vi "Teleop.vi"(10 "Match Info":T1={"Autonomous Elapsed Seconds"=0.0, "TeleOp Elapsed Seconds"=0.0, "Disabled Elapsed Seconds"=0.0, "Visited Autonomous"=FALSE, "Visited TeleOp"=FALSE, "Visited Disabled"=FALSE, "Autonomous Settings"={"Autonomous Style"=enum."Independent", "VI Refnum"=refnum}}, 11 "Call Context":T2) -> ()   [LabVIEW 2014]
doc: "This VI is called for each TeleOp packet received from the DS where the robot is not disabled. It is often used to read from the joysticks and update I/O or to update setpoints for timed control loops. It should complete and return within 20 milliseconds or it may miss DS packets."
uses:
  <vilib>/Rock Robotics/WPI/DriverStation/WPI_DriverStationDerivedRobotMode.ctl
  <vilib>/Rock Robotics/WPI/DriverStation/WPI_DriverStationMatch Info.ctl
  <vilib>/Rock Robotics/Network Tables/SD Read Boolean.vi
  <vilib>/Rock Robotics/Network Tables/SD Read Number.vi
  <vilib>/Rock Robotics/WPI/RobotDrive/WPI_RobotDriveGetSetRefNum.vi
  <vilib>/Rock Robotics/WPI/Joystick/WPI_JoystickGetSetRefNum.vi
  <vilib>/Rock Robotics/Network Tables/SD Write Boolean Array.vi
  <vilib>/Rock Robotics/Network Tables/SD Write Numeric Array.vi
  <vilib>/Rock Robotics/WPI/Solenoid/Deprecated/WPI_SolenoidSetBool.vi
panel:
  in  "Numeric":dbl
  out "2":dbl
  out "9":dbl
  out "8":dbl
  out "Sample Slider 0":dbl(slide) scale=0.0..5.0
  out "Sample Boolean 1":bool
  out "Sample Boolean 0":bool
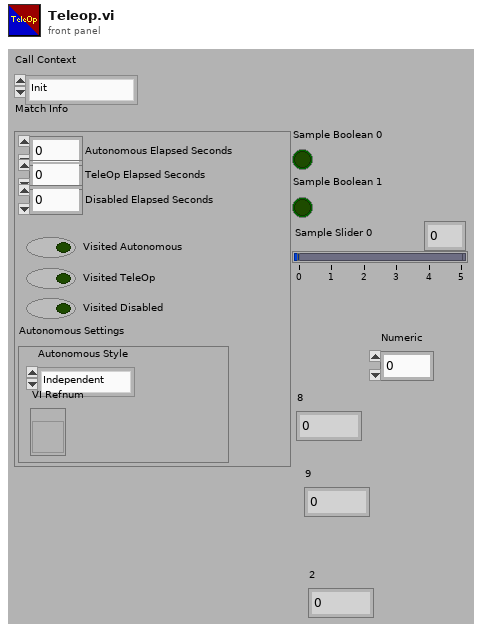
[diagram p1: front panel]
types:
  T1 = typedef "WPI_DriverStationMatch Info.ctl" = cluster{"Autonomous Elapsed Seconds":dbl, "TeleOp Elapsed Seconds":dbl, "Disabled Elapsed Seconds":dbl, "Visited Autonomous":bool, "Visited TeleOp":bool, "Visited Disabled":bool, "Autonomous Settings":cluster{"Autonomous Style":enum16{"Iterative", "Independent"}, "VI Refnum":refnum<vi>}}
  T2 = typedef "WPI_DriverStationDerivedRobotMode.ctl" = enum16{"Init", "Execute", "Stop"}
  T3 = typedef "WPI_JoystickDevRef.ctl" = cluster{"Device":T4}
  T4 = typedef "WPI_JoystickDeviceEnum.ctl" = enum16{"USB 0", "USB 1", "USB 2", "USB 3", "USB 4", "USB 5"}
  T5 = typedef "WPI_RobotDriveDevRef.ctl" = cluster{"DevStatus":errorcluster, "Motors[]":T6[], "Square Inputs":bool, "Max Output":dbl}
  T6 = typedef "WPI_MotorControlDeviceRef.ctl" = cluster{"DeviceStatus":errorcluster, "Type":T7, "PWM":cluster{"Controller":T8, "PWM Channel":T9, "DeadBand":T10}, "CAN":cluster{"Device Number":u8, "Control Mode":T11, "Semaphore":T12, "Max Vout":dbl, "TalonSRX Control Mode":T13}, "Invert":bool, "TransformRef":T14, "InvTransformRef":T14}
  T7 = typedef "WPI_MotorControlType.ctl" = enum16{"PWM", "CAN", "CANTalonSRX"}
  T8 = typedef "FPGA_TypedefDigitalModule.ctl" = enum16{"Controller 1"}
  T9 = typedef "FPGA_DIOPWMChannel.ctl" = enum8{"PWM 0", "PWM 1", "PWM 2", "PWM 3", "PWM 4", "PWM 5", "PWM 6", "PWM 7", "PWM 8", "PWM 9", "PWM MXP 0", "PWM MXP 1", "PWM MXP 2", "PWM MXP 3", "PWM MXP 4", "PWM MXP 5", "PWM MXP 6", "PWM MXP 7", "PWM MXP 8", "PWM MXP 9", "Invalid"}
  T10 = typedef "WPI_PWMDeadband.ctl" = cluster{"Name":string, "maxPositivePwm":i32, "minPositivePwm":i32, "centerPwm":i32, "maxNegativePwm":i32, "minNegativePwm":i32, "angularRange":u16}
  T11 = typedef "WPI_CANJaguar_ControlMode.ctl" = enum8{"Percent VBus", "Current", "Speed", "Position", "Voltage"}
  T12 = typedef "Semaphore RefNum" = refnum<k1>
  T13 = typedef "WPI_CANTalonSRX_APIControlMode.ctl" = enum8{"Percent VBus", "Speed", "Position", "Slave", "Unchanged / Invalid"}
  T14 = typedef "WPI_PWMTransform_ConPane.ctl" = refnum<vi>
  T15 = cluster{"Buttons[0]":bool, "Buttons[1]":bool, "Buttons[2]":bool, "Buttons[3]":bool, "Buttons[4]":bool, "Buttons[5]":bool, "Buttons[6]":bool, "Buttons[7]":bool, "Buttons[8]":bool}
  T16 = cluster{"Axes[0]":dbl, "Axes[1]":dbl, "Axes[2]":dbl, "Axes[3]":dbl, "Axes[4]":dbl, "Axes[5]":dbl, "Axes[6]":dbl, "Axes[7]":dbl, "Axes[8]":dbl}
  T17 = typedef "WPI_SolenoidDevRef.ctl" = cluster{"DevStatus":errorcluster, "Pneumatics Control Module":u8, "Forward Solenoid Channel":T18, "Reverse Solenoid Channel":T18}
  T18 = typedef "WPI_SolenoidChannel.ctl" = enum8{"Solenoid 0", "Solenoid 1", "Solenoid 2", "Solenoid 3", "Solenoid 4", "Solenoid 5", "Solenoid 6", "Solenoid 7", "Invalid"}
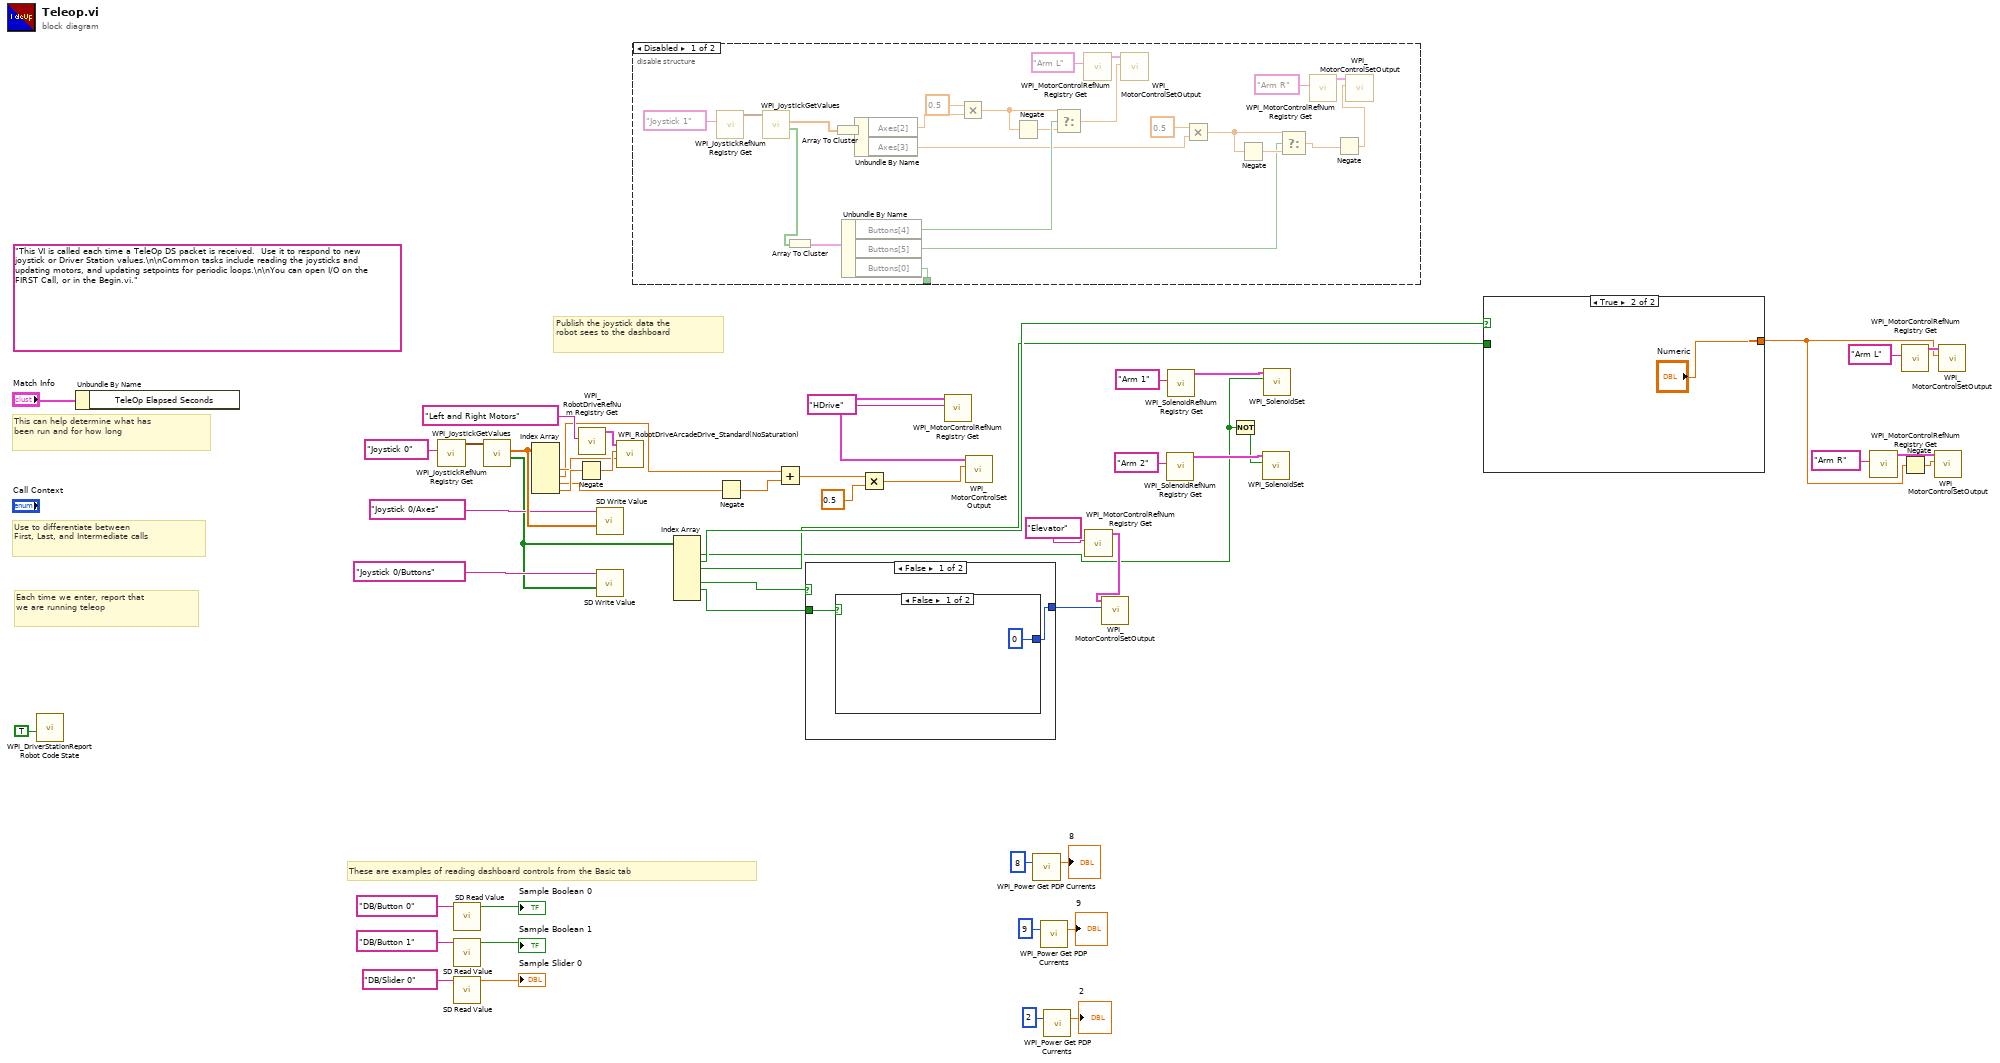
[diagram p0: block diagram]
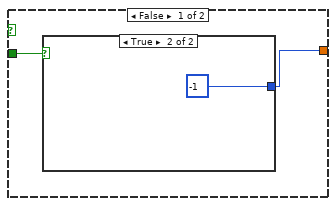
[diagram p3: hidden frame]
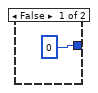
[diagram p4: hidden frame]
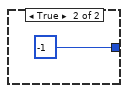
[diagram p5: hidden frame]
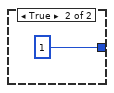
[diagram p6: hidden frame]
diagram:
  (unwired) "This VI is called each time a TeleOp DS packet is received.  Use it to respond to new joystick or Driver Station values.\n\nCommon tasks include reading the joysticks and updating motors, and updating setpoints for periodic loops.\n\nYou can open I/O on the FIRST Call, or in the Begin.vi."
  # "Publish the joystick data the\nrobot sees to the dashboard"
  # "These are examples of reading dashboard controls from the Basic tab"
  # "Each time we enter, report that\nwe are running teleop"
  # "Use to differentiate between\nFirst, Last, and Intermediate calls"
  # "This can help determine what has\nbeen run and for how long"
  n1 = call <vilib>:"WPI_DriverStationReport Robot Code State.vi"("TeleOp"=TRUE ("Autonomous")) -> ()  [unwired: 10 in, 1 out]
  n2 = Unbundle By Name("Match Info") -> ()  [unwired: 1 out]
  n3 = call <vilib>:"WPI_JoystickRefNum Registry Get.vi"("refnum name"="Joystick 0") -> ("JoystickDevRef"=w37:T3)  [unwired: 1 in, 9 out]
  n4 = call-poly <vilib>:"SD Read Value.vi"("Name"="DB/Button 0" ("refnum name")) -> ("Boolean"=→"Sample Boolean 0":bool)  [unwired: 8 in, 2 out]
  n5 = call-poly <vilib>:"SD Read Value.vi"("Name"="DB/Button 1" ("refnum name")) -> ("Boolean"=→"Sample Boolean 1":bool)  [unwired: 8 in, 2 out]
  n6 = call-poly <vilib>:"SD Read Value.vi"("Name"="DB/Slider 0" ("refnum name")) -> ("Numeric"=→"Sample Slider 0":dbl)  [unwired: 8 in, 2 out]
  n7 = call <vilib>:"WPI_JoystickGetValues.vi"("JoystickDevRef"=w37) -> ("Buttons"=w29:bool[], "Axes"=w41:dbl[])  [unwired: 6 in, 3 out]
  n8 = Index Array(array=w41) -> (element #2=w42:dbl, element #3=w33:dbl, element #4=w34:dbl, element #5=w44:dbl)  [unwired: 5 in, 1 out]
  n9 = Negate(x=w44) -> (-x=w43:dbl)
  n10 = call <vilib>:"WPI_RobotDriveRefNum Registry Get.vi"("refnum name"="Left and Right Motors") -> ("RobotDriveDevRef"=w40:T5)  [unwired: 1 in, 9 out]
  n11 = call-poly <vilib>:"SD Write Value.vi"("Numeric Array"=w41, "Name"="Joystick 0/Axes") -> ()  [unwired: 8 in, 2 out]
  n12 = call-poly <vilib>:"SD Write Value.vi"("Boolean Array"=w29, "Name"="Joystick 0/Buttons") -> ()  [unwired: 8 in, 2 out]
  n13 = call <vilib>:"WPI_RobotDriveArcadeDrive_Standard(NoSaturation).vi"("Y axis value"=w42, "X axis value"=w43, "RobotDriveDevRef"=w40) -> ()  [unwired: 1 in, 8 out]
  n14 = disable-structure shown="Disabled" {
    disable-tunnel: [w70 _] -> _
    frame Disabled {
      n15 = call <vilib>:"WPI_JoystickRefNum Registry Get.vi"("refnum name"="Joystick 1") -> ("JoystickDevRef"=w75:T3)  [unwired: 1 in, 9 out]
      n16 = call <vilib>:"WPI_JoystickGetValues.vi"("JoystickDevRef"=w75) -> ("Buttons"=w73:bool[], "Axes"=w71:dbl[])  [unwired: 6 in, 3 out]
      n17 = Array To Cluster(array=w73) -> (cluster=w74:T15)
      n18 = Array To Cluster(array=w71) -> (cluster=w72:T16)
      n19 = Unbundle By Name(w74) -> ("Buttons[4]"=w67:bool, "Buttons[5]"=w57:bool, "Buttons[0]"=w70:bool)
      n20 = Unbundle By Name(w72) -> ("Axes[2]"=w65:dbl, "Axes[3]"=w56:dbl)
      n21 = Multiply(x=0.5, y=w65) -> (x*y=w62:dbl)
      n22 = Negate(x=w62) -> (-x=w63:dbl)
      n23 = Select(t=w62, s=w67, f=w63) -> (s? t:f=w66:dbl)
      n24 = call <vilib>:"WPI_MotorControlRefNum Registry Get.vi"("refnum name"="Arm L") -> ("MotorControlDevRef"=w68:T6)  [unwired: 9 in, 1 out]
      n25 = call <vilib>:"WPI_MotorControlSetOutput.vi"("Output"=w66, "MotorControlDevRef"=w68) -> ()  [unwired: 7 in, 3 out]
      n26 = Multiply(x=0.5, y=w56) -> (x*y=w61:dbl)
      n27 = Negate(x=w61) -> (-x=w60:dbl)
      n28 = Select(t=w61, s=w57, f=w60) -> (s? t:f=w55:dbl)
      n29 = call <vilib>:"WPI_MotorControlRefNum Registry Get.vi"("refnum name"="Arm R") -> ("MotorControlDevRef"=w53:T6)  [unwired: 9 in, 1 out]
      n30 = Negate(x=w55) -> (-x=w54:dbl)
      n31 = call <vilib>:"WPI_MotorControlSetOutput.vi"("Output"=w54, "MotorControlDevRef"=w53) -> ()  [unwired: 7 in, 3 out]
    }
    frame Enabled {
    }
  }
  n32 = Index Array(array=w29) -> (element #1=w3:bool, element #2=w11:bool, element #3=w10:bool, element #5=w27:bool, element #6=w24:bool)  [unwired: 7 in, 2 out]
  n33 = Negate(x=w34) -> (-x=w32:dbl)
  n34 = Add(x=w33, y=w32) -> (x+y=w23:dbl)
  n35 = case shown="False" w27 {
    tunnel: [w77 1] -> w25
    tunnel: w24 -> [w78 _]
    frame False {
      n36 = case shown="False" w78 {
        tunnel: [0 -1] -> w77
        frame False {
        }
        frame True {
        }
      }
    }
    frame True {
    }
  }
  n37 = Multiply(x=w23, y=0.5) -> (x*y=w22:dbl)
  n38 = call <vilib>:"WPI_MotorControlRefNum Registry Get.vi"("refnum name"="HDrive") -> ("MotorControlDevRef"=w31:T6)  [unwired: 9 in, 1 out]
  n39 = call <vilib>:"WPI_MotorControlSetOutput.vi"("Output"=w22, "MotorControlDevRef"=w31) -> ()  [unwired: 7 in, 3 out]
  n40 = call <vilib>:"WPI_Power Get PDP Currents.vi"("PDP Channel"=8) -> ("current (A)"=→"8":dbl)  [unwired: 12 in, 2 out]
  n41 = call <vilib>:"WPI_Power Get PDP Currents.vi"("PDP Channel"=9) -> ("current (A)"=→"9":dbl)  [unwired: 12 in, 2 out]
  n42 = call <vilib>:"WPI_Power Get PDP Currents.vi"("PDP Channel"=2) -> ("current (A)"=→"2":dbl)  [unwired: 12 in, 2 out]
  n43 = call <vilib>:"WPI_MotorControlRefNum Registry Get.vi"("refnum name"="Elevator") -> ("MotorControlDevRef"=w26:T6)  [unwired: 9 in, 1 out]
  n44 = call <vilib>:"WPI_MotorControlSetOutput.vi"("Output"=w25, "MotorControlDevRef"=w26) -> ()  [unwired: 7 in, 3 out]
  n45 = call <vilib>:"WPI_SolenoidRefNum Registry Get.vi"("refnum name"="Arm 2") -> ("SolenoidDevRef"=w17:T17)  [unwired: 9 in, 1 out]
  n46 = call <vilib>:"WPI_SolenoidRefNum Registry Get.vi"("refnum name"="Arm 1") -> ("SolenoidDevRef"=w20:T17)  [unwired: 9 in, 1 out]
  n47 = Not(x=w3) -> (.not. x?=w16:bool)
  n48 = call-poly <vilib>:"WPI_SolenoidSet.vi"("Value"=w16, "SolenoidDevRef"=w17) -> ()  [unwired: 8 in, 2 out]
  n49 = call-poly <vilib>:"WPI_SolenoidSet.vi"("Value"=w3, "SolenoidDevRef"=w20) -> ()  [unwired: 8 in, 2 out]
  n50 = case shown="True" w11 {
    tunnel: [w83 "Numeric"] -> w4
    tunnel: w10 -> [w82 _]
    frame False {
      n51 = case shown="True" w82 {
        tunnel: [0 -1] -> w83
        frame False {
        }
        frame True {
        }
      }
    }
    frame True {
    }
  }
  n52 = call <vilib>:"WPI_MotorControlRefNum Registry Get.vi"("refnum name"="Arm R") -> ("MotorControlDevRef"=w8:T6)  [unwired: 9 in, 1 out]
  n53 = call <vilib>:"WPI_MotorControlRefNum Registry Get.vi"("refnum name"="Arm L") -> ("MotorControlDevRef"=w9:T6)  [unwired: 9 in, 1 out]
  n54 = Negate(x=w4) -> (-x=w7:dbl)
  n55 = call <vilib>:"WPI_MotorControlSetOutput.vi"("Output"=w7, "MotorControlDevRef"=w8) -> ()  [unwired: 7 in, 3 out]
  n56 = call <vilib>:"WPI_MotorControlSetOutput.vi"("Output"=w4, "MotorControlDevRef"=w9) -> ()  [unwired: 7 in, 3 out]
